vi "Get Outputs.vi"(8 "error in (no error)":errorcluster, 10 "Names":string[](array[string]), 11 "Node in":refnum<vi>) -> (0 "error out":errorcluster, 2 "Outputs":refnum<vi>[](array[refnum]), 3 "Node out":refnum<vi>)   [LabVIEW 2015, in "Scripting.lvlib"]
doc: "<B>bold</B>"
uses:
  Scripting.lvlib
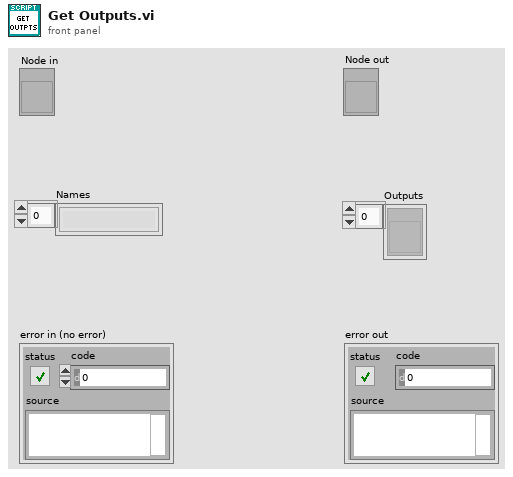
[diagram p1: front panel]
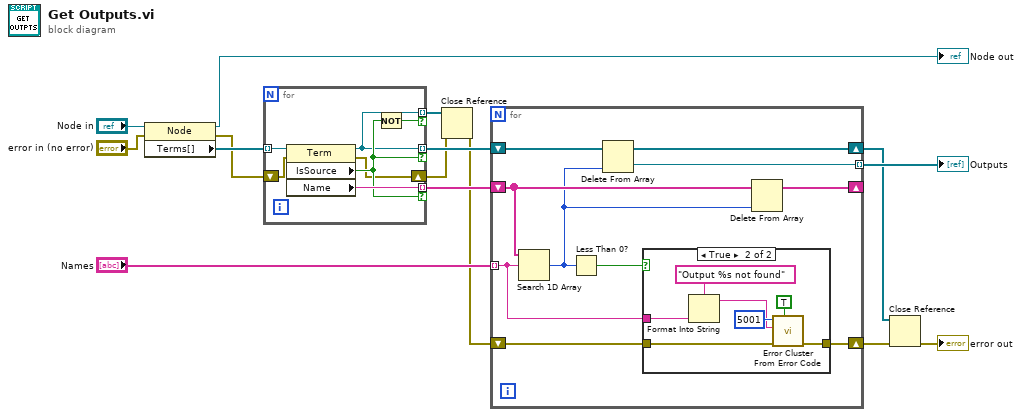
[diagram p0: block diagram]
diagram:
  n1 = property class="Node"(reference="Node in", error in="error in (no error)") -> (reference out=→"Node out":refnum<vi>, error out=w9:errorcluster, "Terms[]"=w13:refnum<vi>[])
  n2 = for {
    tunnel: w13 -> [w22] mode=indexing
    tunnel: [w18] -> w12 mode=indexing if=w19
    tunnel: [w21] -> w11 mode=indexing if=w19
    tunnel: [w18] -> w6 mode=indexing if=w16
    shift-right: [w17] -> w5
    shift-left: w9 -> [w20]
    n3 = property class="Term"(reference=w22, error in=w20) -> (reference out=w18:refnum<vi>, error out=w17:errorcluster, "IsSource"=w19:bool, "Name"=w21:string)
    n4 = Not(x=w19) -> (.not. x?=w16:bool)
  }
  n5 = Close Reference(reference=w6, error in (no error)=w5) -> (error out=w4:errorcluster)
  n6 = for {
    tunnel: "Names" -> [w29] mode=indexing
    shift-right: [w25] -> w2
    shift-left: w4 -> [w30]
    shift-right: [w26] -> _
    shift-left: w11 -> [w28]
    tunnel: [w24] -> w7 mode=indexing
    shift-right: [w23] -> w3
    shift-left: w12 -> [w32]
    n7 = Search 1D Array(1D array=w28, element=w29) -> (index of element=w27:i32)  [unwired: 1 in]
    n8 = Less Than 0?(x=w27) -> (x < 0?=w31:bool)
    n9 = Delete From Array(array=w32, index=w27) -> (deleted portion=w24:refnum<vi>, array with subset deleted=w23:refnum<vi>[])  [unwired: 1 in]
    n10 = case shown="True" w31 {
      tunnel: w30 -> [w33 w39]
      tunnel: w29 -> [_ w37]
      tunnel: [w33 w34] -> w25
      frame False {
      }
      frame True {
        n11 = Format Into String(format string="Output %s not found", w37) -> (resulting string=w36:string)  [unwired: 2 in, 1 out]
        n12 = call <vilib>:"Error Cluster From Error Code.vi"("show call chain? (False)"=TRUE, "error in (no error)"=w39, "error message (\"\")"=w36, "error code (0)"=5001) -> ("error out"=w34:errorcluster)  [unwired: 5 in]
      }
    }
    n13 = Delete From Array(array=w28, index=w27) -> (array with subset deleted=w26:string[])  [unwired: 1 in, 1 out]
  }
  "Outputs" <- w7
  n14 = Close Reference(reference=w3, error in (no error)=w2) -> (error out=→"error out":errorcluster)
